vi "Update LED Cards.vi"(8 "error in (no error)":errorcluster, 10 "Bitfile Info":T1, 11 "Device Ref in":T2 format="%.0x") -> (0 "error out":errorcluster)   [LabVIEW 2014, in "SLSC configuration System Explorer.lvlib"]
uses:
  SLSC configuration System Explorer.lvlib
  <vilib>/NI Veristand/Custom Device API/Custom Device Item Ref.ctl
  Type Defs/SLSC Bitfile Info.ctl
  Shared/Constants.vi
  Shared/SLSC configuration Shared.lvlib
  <vilib>/NI Veristand/Custom Device API/Custom Device API.lvlib
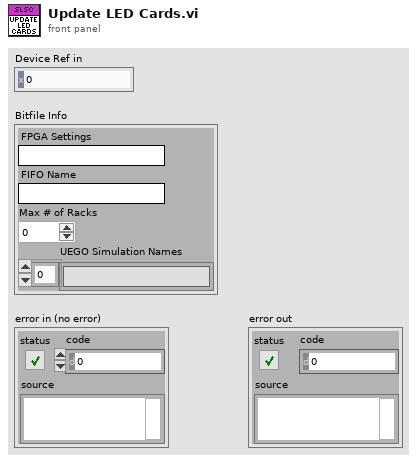
[diagram p1: front panel]
types:
  T1 = typedef "SLSC configuration System Explorer.lvlib/SLSC Bitfile Info.ctl" = cluster{"FPGA Settings":string, "FIFO Name":string, "Max # of Racks":u8, "UEGO Simulation Names":string[]}
  T2 = typedef "Custom Device API.lvlib/Custom Device Item Ref.ctl" = u64
  T3 = typedef "SLSC configuration Shared.lvlib/Card Position.ctl" = cluster{"Rack #":u8, "Slot #":T4}
  T4 = typedef "SLSC configuration Shared.lvlib/Slot #.ctl" = u8
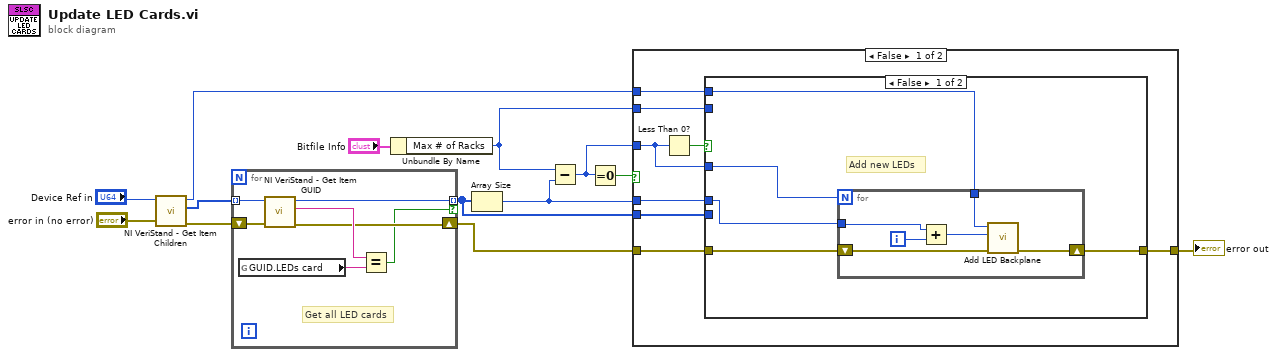
[diagram p0: block diagram]
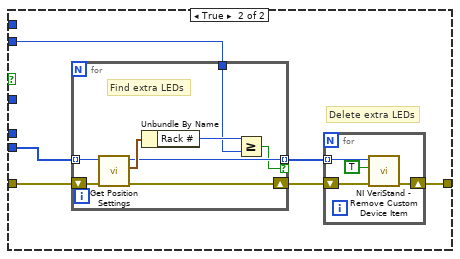
[diagram p2: hidden frame]
diagram:
  n1 = call <vilib>:"NI VeriStand - Get Item Children.vi"("error in (no error)"="error in (no error)", "Item Ref in"="Device Ref in") -> ("error out"=w3:errorcluster, "Child Refs"=w4:T2[], "Item Ref out"=w5:T2)  [unwired: 6 in, 1 out]
  n2 = for {
    shift-right: [w17] -> w9
    shift-left: w3 -> [w19]
    tunnel: [w16] -> w10 mode=indexing if=w15
    tunnel: w4 -> [w14] mode=indexing
    # "Get all LED cards"
    n3 = global read "Constants.vi" "GUID.LEDs card"() -> (w20:string)
    n4 = call <vilib>:"NI VeriStand - Get Item GUID.vi"("error in (no error)"=w19, "Item Ref in"=w14) -> ("error out"=w17:errorcluster, "GUID"=w18:string, "Item Ref out"=w16:T2)  [unwired: 7 in]
    n5 = Equal?(x=w18, y=w20) -> (x = y?=w15:bool)
  }
  n6 = Unbundle By Name("Bitfile Info") -> ("Max # of Racks"=w2:u8)
  n7 = Array Size(array=w10) -> (size(s)=w1:i32)
  n8 = Subtract(x=w2, y=w1) -> (x-y=w11:i32)
  n9 = Equal To 0?(x=w11) -> (x = 0?=w12:bool)
  n10 = case shown="False" w12 {
    tunnel: w11 -> [w27 _]
    tunnel: w10 -> [w28 _]
    tunnel: w9 -> [w25 w58]
    tunnel: [w24 w58] -> w8
    tunnel: w5 -> [w23 _]
    tunnel: w2 -> [w22 _]
    tunnel: w1 -> [w21 _]
    frame False {
      n11 = Less Than 0?(x=w27) -> (x < 0?=w26:bool)
      n12 = case shown="False" w26 {
        tunnel: w28 -> [_ w43]
        tunnel: w27 -> [w30 _]
        tunnel: w25 -> [w33 w44]
        tunnel: [w32 w45] -> w24
        tunnel: w23 -> [w31 _]
        tunnel: w22 -> [_ w42]
        tunnel: w21 -> [w29 _]
        frame False {
          # "Add new LEDs"
          n13 = for {
            N: w30 -> [_]
            tunnel: w31 -> [w39]
            shift-right: [w37] -> w32
            shift-left: w33 -> [w38]
            tunnel: w29 -> [w35]
            i -> [w36]
            n14 = Add(x=w35, y=w36) -> (x+y=w34:i32)
            n15 = call "Add LED Backplane.vi"("error in (no error)"=w38, "Rack #"=w34, "Node Ptr"=w39) -> ("error out"=w37:errorcluster)  [unwired: 8 in]
          }
        }
        frame True {
          # "Delete extra LEDs"
          n16 = for {
            tunnel: w43 -> [w51] mode=indexing
            tunnel: [w50] -> w40 mode=indexing if=w47
            tunnel: w42 -> [w48]
            shift-right: [w46] -> w41
            shift-left: w44 -> [w52]
            # "Find extra LEDs"
            n17 = call "Get Position Settings.vi"("error in (no error)"=w52, "Item Ref in"=w51) -> ("error out"=w46:errorcluster, "Card Position"=w53:T3, "Item Ref out"=w50:T2)  [unwired: 7 in]
            n18 = Unbundle By Name(w53) -> ("Rack #"=w49:u8)
            n19 = Greater Or Equal?(x=w49, y=w48) -> (x >= y?=w47:bool)
          }
          n20 = for {
            shift-right: [w55] -> w45
            shift-left: w41 -> [w56]
            tunnel: w40 -> [w54] mode=indexing
            n21 = call <vilib>:"NI VeriStand - Remove Custom Device Item.vi"("error in (no error)"=w56, "Force Delete (F)"=TRUE, "Item Ref in"=w54) -> ("error out"=w55:errorcluster)  [unwired: 7 in, 1 out]
          }
        }
      }
    }
    frame True {
      # "All LEDs accounted for"
    }
  }
  "error out" <- w8
